vi "Plasma.vi"(8 "Periods2":i32, 9 "Periods1":i32, 10 "N2":i32, 11 "N1":i32) -> (1 "Array":dbl[][](array[numeric]), 2 "N2 2":i32, 3 "N1 out":i32)   [LabVIEW 2014]
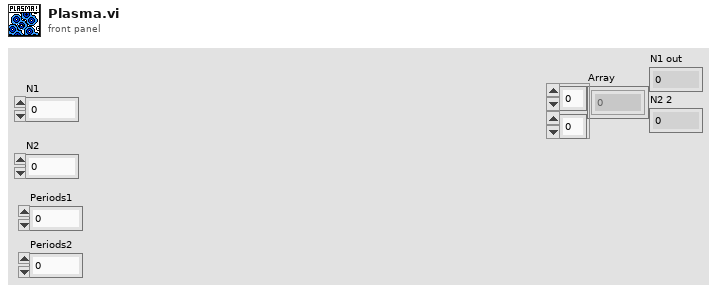
[diagram p1: front panel]
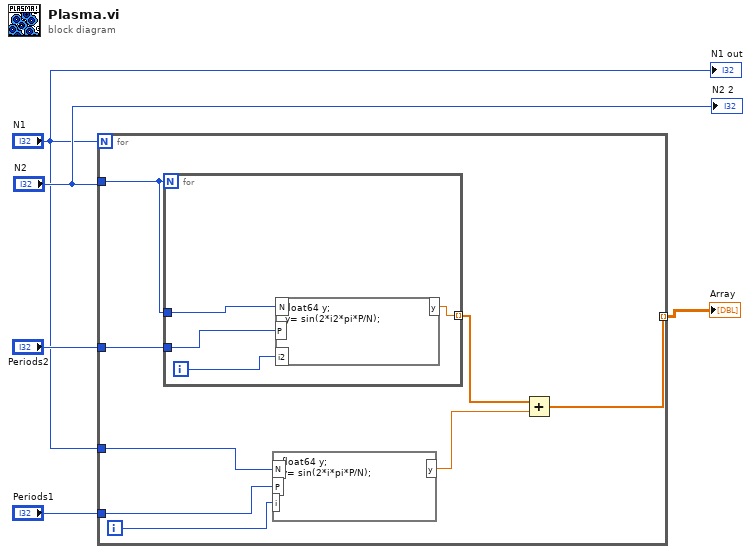
[diagram p0: block diagram]
diagram:
  n1 = for {
    N: "N1" -> [_]
    tunnel: "N1" -> [w9]
    tunnel: "N2" -> [w13]
    tunnel: "Periods2" -> [w12]
    tunnel: "Periods1" -> [w8]
    tunnel: [w10] -> w1 mode=indexing
    i -> [w6]
    n2 = for {
      N: w13 -> [_]
      tunnel: w13 -> [w17]
      tunnel: w12 -> [w16]
      tunnel: [w14] -> w11 mode=indexing
      i -> [w15]
      n3 = formula code="float64 y;\ny= sin(2*i2*pi*P/N);" ("Formelknoten")("N"=w17, "P"=w16, "i2"=w15) -> ("y"=w14:dbl)
    }
    n4 = formula code="float64 y;\ny= sin(2*i*pi*P/N);" ("Formelknoten")("N"=w9, "P"=w8, "i"=w6) -> ("y"=w7:dbl)
    n5 = Add(x=w11, y=w7) -> (x+y=w10:dbl[])
  }
  "Array" <- w1
  "N1 out" <- "N1"
  "N2 2" <- "N2"
